vi "Dashboard Main.vi"() -> ()   [LabVIEW 2015]
uses:
  <vilib>/Utility/miscctls.llb/LVRowAndColumnTypeDef.ctl
  <vilib>/event_ctls.llb/eventvkey.ctl
  <vilib>/Rock Robotics/WPI/Dashboard/WPI_DashboardLogging Global.vi
  <vilib>/Rock Robotics/Network Tables/NT Read Numeric Array.vi
  <vilib>/Rock Robotics/Network Tables/NT Read Boolean.vi
  <vilib>/Utility/config.llb/Write Key (String).vi
  <vilib>/Utility/config.llb/Write Key (I32).vi
  <vilib>/Utility/config.llb/NI_LVConfig.lvlib
panel:
  in  "TCP":refnum<k5>
  in  "Rec Mode":enum32{"Stop", "Record", "Playback"}(radio)
  in  "Vision":u16(ring) items=["Camera Off", "USB Camera SW", "USB Camera HW", "IP Camera"]
  out "Camera IP":string
  out "Image Message":string="Timeout in Camera Communications"
  in  "Dashboard Tab":T1(tab)
  out "Voltage":dbl
  out "Current":dbl
  out "Pivot Outputs":cluster{"Numeric":dbl, "Numeric":dbl}(graph)
  out "Shooter":bool
  out "Fire":bool
  out "IntakePivot":bool
  out "IntakeRoller":bool
  out "Angle":dbl(slide) scale=-40.0..55.0
  in  "Select Auto":string(combo)
  out "NT Connection":bool
  in  "Camera Settings":T2={"Frame Rate"=30, "Compression"=30, "Size"=1} {"Frame Rate" scale=1.0..30.0; "Size" items=["640x480", "320x240", "160x120"]}
  out "MotorChart R":cluster{"Numeric":dbl, "Numeric":dbl}(graph)
  out "MotorChart L":T3(graph)
  out "MotorSliders R":cluster{"MotorSlide1":dbl, "MotorSlide2":dbl} {"MotorSlide2" scale=-1.0..1.0 scale format="%#_2e"; "MotorSlide1" scale=-1.0..1.0 scale format="%#_2e"}
  out "MotorSliders L":T4 {"MotorSlide4 2" scale=0.0..14.0 scale format="%#_2e"; "MotorSlide2" scale=-1.0..1.0 scale format="%#_2e"; "MotorSlide1" scale=-1.0..1.0 scale format="%#_2e"}
  out "JS1 Z":dbl(slide) scale=-1.0..1.0 scale format="%#_2e"
  out "JS1 Graph":cluster{"X":dbl, "Y":dbl}[](graph)
  out "JS1 Buttons":T5
  out "JS2 Z":dbl(slide) scale=-1.0..1.0 scale format="%#_2e"
  out "JS2 Graph":cluster{"X":dbl, "Y":dbl}[](graph)
  out "JS2 Buttons":T5
  out "Mode":T6(ring)=enum."Auto Disabled"
  in  "DB Camera Config":bool
  out "fps":dbl format="%#.1g"
  out "Mbps":dbl format="%#.1g"
  out "Mbps LED":bool
  in  "DB/String 9":string
  in  "DB/String 8":string
  in  "DB/String 7":string
  in  "DB/String 6":string
  in  "DB/String 5":string
  in  "DB/String 4":string
  in  "DB/String 3":string
  in  "DB/String 2":string
  in  "DB/String 1":string
  in  "DB/String 0":string
  in  "DB/Slider 0":dbl(slide) scale=0.0..5.0
  in  "DB/Slider 1":dbl(slide) scale=0.0..5.0
  in  "DB/Slider 2":dbl(slide) scale=0.0..5.0
  in  "DB/Slider 3":dbl(slide) scale=0.0..5.0
  out "DB/LED 3":bool
  out "DB/LED 2":bool
  out "DB/LED 1":bool
  out "DB/LED 0":bool
  in  "DB/Button 3":bool
  in  "DB/Button 2":bool
  in  "DB/Button 1":bool
  in  "DB/Button 0":bool caption="New Name"
  in  "Test Slider":dbl(slide) scale=0.0..100.0 scale format="%#_3g"
  in  "On/Off":bool caption="Solenoid"
  in  "Test Name":u16(ring) items=["Select the test to run..."]
  in  "Test Tree":string(tree)
  in  "Motor":cluster{"Value":dbl, "Enable":bool} {"Value" scale=-1.0..1.0 scale format="%#_3g"}
  out "Progress":T7 {"Test Progress" scale=0.0..100.0}
  in  "Rev/Fwd":cluster{"Forward":bool, "Reverse":bool}
  in  "Test Ring":u16(ring) items=["Monochrome", "Color"]
  out "Cmd Status":string
  in  "Execute Command":bool
  in  "Command Params":string[][](table)
  in  "Command Selection":i32(listbox)
  in  "CheckList":i32(listbox)
  out "Tree":string(tree)
  out "Camera Image":T8(plugin-control)
  out "Background":bool
  # "Left"
  # "Front"
  # "Right"
  # "Battery"
  # "This tab is a great place for autonomous settings and robot-specific values.\nPlace controls and indicators inside this tab and match name to\nDashboard Variables on robot. You can also delete this comment."
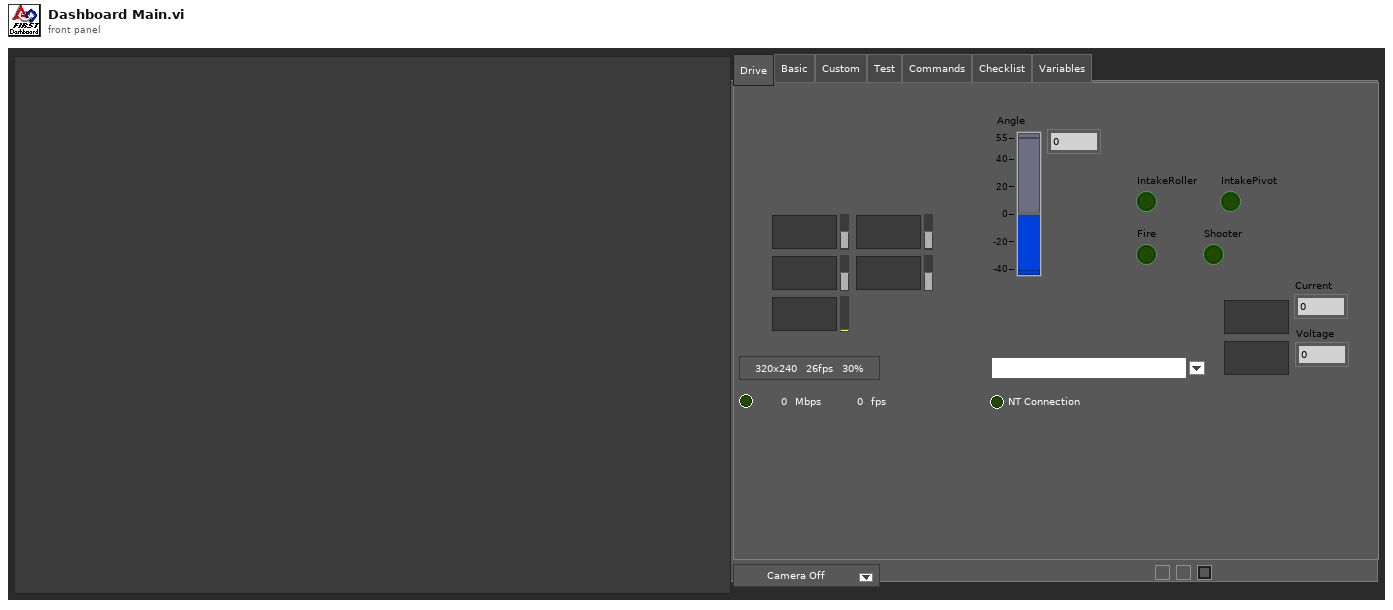
[diagram p1: front panel]
types:
  T1 = enum32{"Drive", "Basic", "Custom", "Test", "Commands", "Checklist", "Variables"}
  T2 = cluster{"Frame Rate":i32, "Compression":i32, "Size":u16}
  T3 = cluster{"Numeric":dbl, "Numeric":dbl, "Battery V":dbl}
  T4 = cluster{"MotorSlide1":dbl, "MotorSlide2":dbl, "MotorSlide4 2":dbl}
  T5 = cluster{bool, bool, bool, bool, bool, bool, bool, bool, bool, bool, bool, bool}
  T6 = enum8{"Tele-Op Disabled", "Tele-Op Enabled", "Auto Disabled", "Auto Enabled", "Test Disabled", "Test Enabled", "Disconnected", "No Code", "E-Stop"}
  T7 = cluster{"Test Progress":u8, "Test Progress Text":string}
  T8 = typedef "IMAQ Image.ctl" = refnum<image>
  T9 = cluster{"IDs":cluster{"RPC field ID":u16, "Unique ID":u16}, "String":string}
  T10 = enum32{"Drive", "Basic", "Custom", "Test", "Checklist", "Variables"}
  T11 = typedef "Image Type" = u32
  T12 = cluster{"Camera Image":refnum<vi>, "Dashboard Tab":refnum<vi>, "Background":refnum<vi>, "Vision":refnum<vi>, "Rec Mode":refnum<vi>, "Test Slider":refnum<vi>, "On/Off ":refnum<vi>, "Test Ring":refnum<vi>, "Rev/Fwd":refnum<vi>, "Test Name":refnum<vi>, "Motor":refnum<vi>, "Progress":refnum<vi>, "CheckList":refnum<vi>, "Tree":refnum<vi>, "Test Tree":refnum<vi>, "Command Params":refnum<vi>, "Command Selection":refnum<vi>, "Execute Command":refnum<vi>, "Cmd Status":refnum<vi>}
  T13 = cluster{"Error Strings":string, "Disable Counts":cluster{u16, u16}, "Rail Faults":cluster{u16, u16, u16}, "Robot IP":string, "DB Mode":u8, "Event Info":cluster{"Name":string, "Type":u8, "Number":u16, "Replay":u8}, "Camera Addr":string}
  T14 = cluster{"Storage":cluster{"Disk Free":u64, "RAM Block":u32, "RAM free":u32}, "CPU Utilization":cluster{"CPU % ISR":sgl, "CPU % Time Crit":sgl, "CPU % Timed Str":sgl, "CPU % High":sgl, "CPU % Above":sgl, "CPU % Normal":sgl, "CPU % Low":sgl}, "CAN":cluster{"% Bus Utilization":sgl, "Bus Off Cnt":u32, "TX_FIFO Full Cnt":u32, "Receive Error Cnt":u8, "Transmit Error Cnt":u8}, "HID":cluster{"HID Outputs":u32, "Rumble Low":u16, "Rumble High":u16}[]}
  T15 = cluster{"Status bits":cluster{"Test Mode":bool, "Autonomous":bool, "Enabled":bool, "Code Start":bool, "Brownout":bool, "Reserved 2":bool, "Reserved 3":bool, "E-Stop":bool}, "Code Trace":cluster{"Disabled":bool, "TeleOp":bool, "Auto":bool, "Test":bool}, "Controller Type":enum16{"unknown", "cRIO", "roboRio"}, "Code?":enum16{"unknown", "noCode", "code"}, "Battery V":dbl}
  T16 = cluster{"Control Bits":cluster{"TestMode":bool, "Autonomous":bool, "Enabled":bool, "FMS Present":bool, bool, bool, bool, "E-Stop":bool}, "Team Station ":u8, "Countdown":sgl, "Joystick Values":cluster{"Axes":dbl[], "Buttons":bool[], "POVs":i16[]}[]}
  T17 = cluster{"Axes":dbl[], "Buttons":bool[], "POVs":i16[]}[]
  T18 = cluster{"Axes":dbl[], "Buttons":bool[], "POVs":i16[]}
  T19 = cluster{"Buttons[0]":bool, "Buttons[1]":bool, "Buttons[2]":bool, "Buttons[3]":bool, "Buttons[4]":bool, "Buttons[5]":bool, "Buttons[6]":bool, "Buttons[7]":bool, "Buttons[8]":bool, "Buttons[9]":bool, "Buttons[10]":bool, "Buttons[11]":bool}
  T20 = typedef "NI_LVConfig.lvlib/Config Data RefNum.ctl" = refnum<k1>
  T21 = cluster{"Operation":enum16{"Update", "Clear"}, "Color Box":u32}[]
  T22 = typedef "eventvkey.ctl" = enum16{"ASCII", "Enter", "Return", "Shift", "Ctrl", "Alt", "Cmd", "Opt", "Caps", "NumLock", "Clear", "Break", "Up", "Down", "Left", "Right", "Insert", "Delete", "Home", "End", "PageUp", "PageDown", "Escape", "Help", "Pause", "ScrollLock", "F1", "F2", "F3", "F4", "F5", "F6", "F7", "F8", "F9", "F10", "F11", "F12", "F13", "F14", "F15", "F16", "F17", "F18", "F19", "F20", "F21", "F22", "F23", "F24", "Play", "VolumeUp", "VolumeDown", "Mute", "Two Byte Char"}
  T23 = cluster{"Image Size":bool, "Image Type":bool, "Pixel Value":bool, "ROI Information":bool, "Zoom Factor":bool}
  T24 = enum8{"Enabled", "Disabled", "Disabled and Grayed Out"}
  T25 = cluster{"Operation":enum16{"Update", "Clear"}, "Color Box":u32}
  T26 = typedef "LVRowAndColumnTypeDef.ctl" = cluster{"Row":i32, "Column":i32}
  T27 = cluster{"Shift":bool, "Ctrl":bool, "Alt":bool, "Cmd":bool, "Opt":bool}
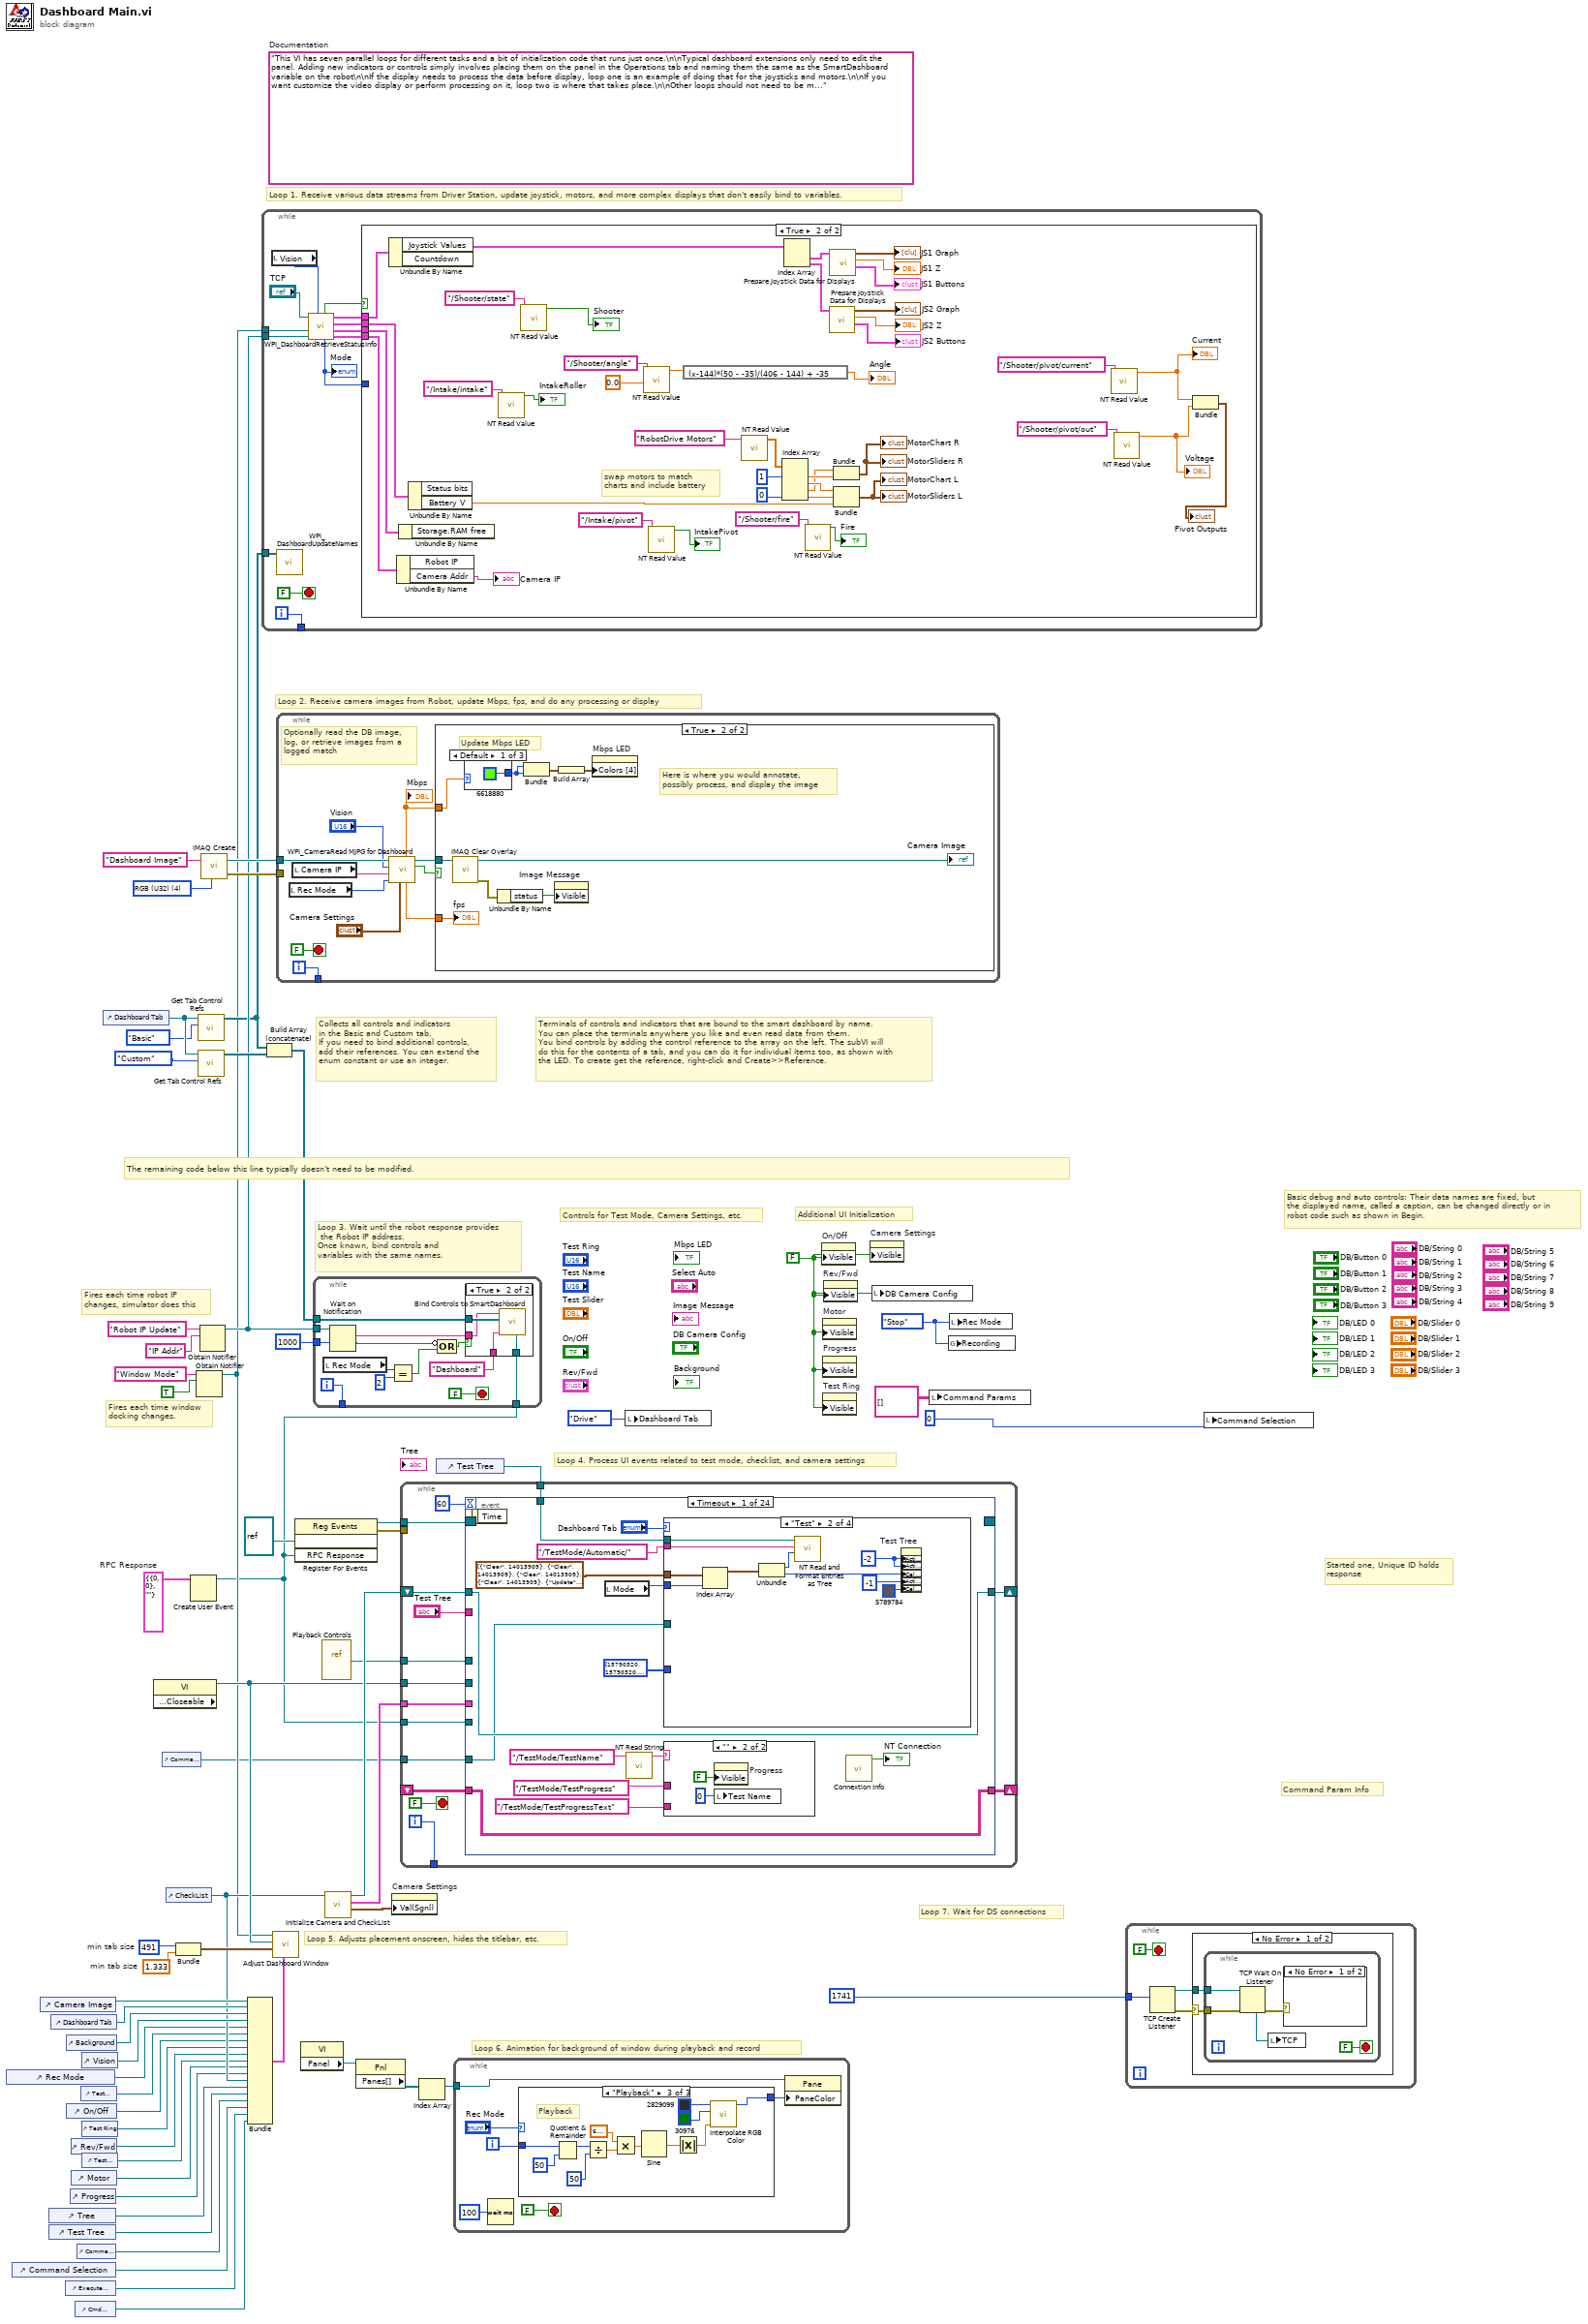
[diagram p0: block diagram]
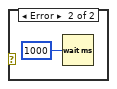
[diagram p2: hidden frame]
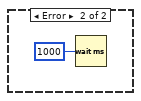
[diagram p3: hidden frame]
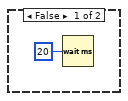
[diagram p4: hidden frame]
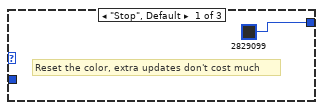
[diagram p5: hidden frame]
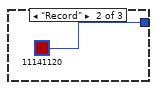
[diagram p6: hidden frame]
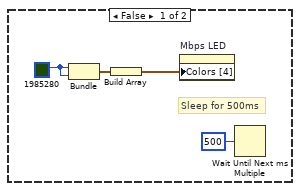
[diagram p8: hidden frame]
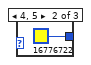
[diagram p9: hidden frame]
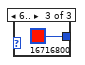
[diagram p10: hidden frame]
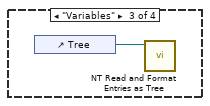
[diagram p12: hidden frame]
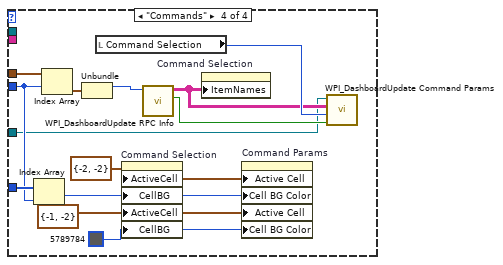
[diagram p13: hidden frame]
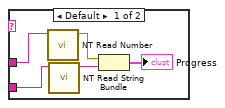
[diagram p14: hidden frame]
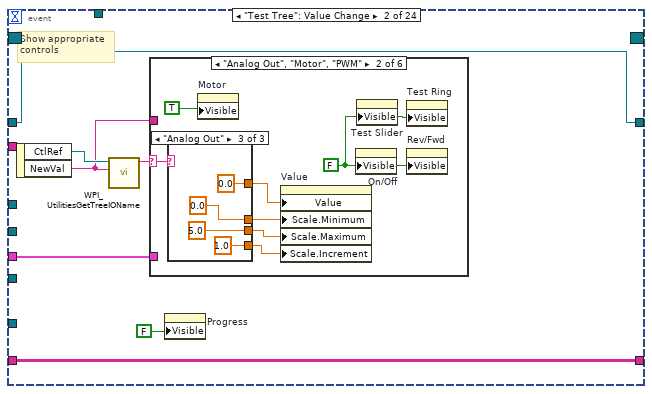
[diagram p15: hidden frame]
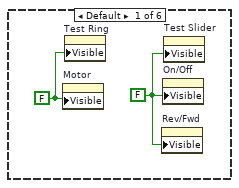
[diagram p16: hidden frame]
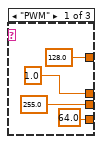
[diagram p17: hidden frame]
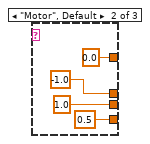
[diagram p18: hidden frame]
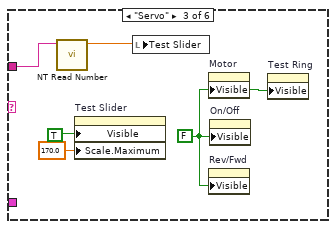
[diagram p19: hidden frame]
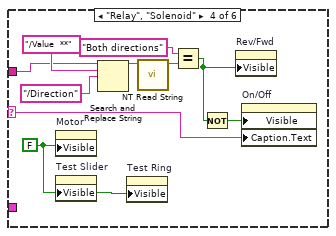
[diagram p20: hidden frame]
diagram:
  w7 = T9 {"IDs"={"RPC field ID"=0, "Unique ID"=0}, "String"=""}  # RPC Response
  w33 = 491  # min tab size
  w32 = 1.333  # min tab size
  w41 = enum32{"Stop", "Record", "Playback"}."Stop" ("Rec Mode")
  w15 = FALSE ("Visible")
  (unwired) "This VI has seven parallel loops for different tasks and a bit of initialization code that runs just once.\n\nTypical dashboard extensions only need to edit the panel. Adding new indicators or controls simply involves placing them on the panel in the Operations tab and naming them the same as the SmartDashboard variable on the robot\n\nIf the display needs to process the data before display, loop one is an example of doing that for the joysticks and motors.\n\nIf you want customize the video display or perform processing on it, loop two is where that takes place.\n\nOther loops should not need to be modified. They are pretty standard, and document the task they perform."  # Documentation
  w61 = T11 4 items=["Grayscale (U8)", "Grayscale (I16)", "Grayscale (SGL)", "Complex (CSG)", "RGB (U32)", "HSL (U32)", "RGB (U64)"] ("Image Type")
  # "Command Param Info"
  # "Started one, Unique ID holds\nresponse"
  # "Loop 7. Wait for DS connections"
  # "Basic debug and auto controls: Their data names are fixed, but\nthe displayed name, called a caption, can be changed directly or in\nrobot code such as shown in Begin."
  # "Controls for Test Mode, Camera Settings, etc."
  # "Additional UI Initialization"
  # "Loop 6. Animation for background of window during playback and record"
  # "Fires each time robot IP\nchanges, simulator does this"
  # "Fires each time window\ndocking changes."
  # "Collects all controls and indicators\nin the Basic and Custom tab.\nIf you need to bind additional controls,\nadd their references. You can extend the\nenum constant or use an integer."
  # "The remaining code below this line typically doesn't need to be modified."
  # "Loop 4. Process UI events related to test mode, checklist, and camera settings"
  # "Terminals of controls and indicators that are bound to the smart dashboard by name.\nYou can place the terminals anywhere you like and even read data from them.\nYou bind controls by adding the control reference to the array on the left. The subVI will\ndo this for the contents of a tab, and you can do it for individual items too, as shown with\nthe LED. To create get the reference, right-click and Create>>Reference."
  # "Loop 3. Wait until the robot response provides\n the Robot IP address.\nOnce known, bind controls and\nvariables with the same names."
  # "Loop 5. Adjusts placement onscreen, hides the titlebar, etc."
  # "Loop 1. Receive various data streams from Driver Station, update joystick, motors, and more complex displays that don't easily bind to variables."
  # "Loop 2. Receive camera images from Robot, update Mbps, fps, and do any processing or display"
  n1 = control-ref of="Rec Mode"() -> (w21:refnum<vi>)
  n2 = control-ref of="Command Selection"() -> (w6:refnum<vi>)
  n3 = control-ref of="Camera Image"() -> (w36:refnum<vi>)
  n4 = control-ref of="Tree"() -> (w25:refnum<vi>)
  n5 = control-ref of="Test Tree"() -> (w24:refnum<vi>)
  n6 = control-ref of="Dashboard Tab"() -> (w35:refnum<vi>)
  n7 = control-ref of="Execute Command"() -> (w8:refnum<vi>)
  n8 = control-ref of="Background"() -> (w30:refnum<vi>)
  n9 = control-ref of="On/Off"() -> (w19:refnum<vi>)
  n10 = control-ref of="Progress"() -> (w16:refnum<vi>)
  n11 = control-ref of="Rev/Fwd"() -> (w17:refnum<vi>)
  n12 = control-ref of="Motor"() -> (w22:refnum<vi>)
  n13 = control-ref of="Cmd Status"() -> (w2:refnum<vi>)
  n14 = control-ref of="Command Params"() -> (w9:refnum<vi>)
  n15 = control-ref of="Test Slider"() -> (w20:refnum<vi>)
  n16 = control-ref of="Vision"() -> (w34:refnum<vi>)
  n17 = control-ref of="Test Ring"() -> (w18:refnum<vi>)
  n18 = control-ref of="Test Name"() -> (w23:refnum<vi>)
  n19 = control-ref of="Dashboard Tab"() -> (w39:refnum<vi>)
  n20 = property class="VI" props=["Front Panel.Closeable"]() -> (reference out=w40:refnum<vi>)  [unwired: 2 in, 2 out]
  n21 = control-ref of="Command Params"() -> (w1:refnum<vi>)
  n22 = control-ref of="CheckList"() -> (w26:refnum<vi>)
  n23 = Bundle("min tab size"=w33, "min tab size"=w32) -> (w31:cluster{"min tab size":i32, "min tab size":dbl})  [unwired: 1 in]
  n24 = Create User Event(user event datatype=w7) -> (user event=w3:refnum<user-event>)  [unwired: 1 in, 1 out]
  n25 = Obtain Notifier(name (unnamed)="Window Mode", notification data type=TRUE) -> (notifier out=w12:refnum<notifier>)  [unwired: 2 in, 2 out]
  n26 = call <vilib>:"Get Tab Control Refs.vi"("Page Index"=T10."Basic" ("Dashboard Tab"), "TabControl in"=w39) -> ("ControlsOnPage"=w13:refnum<vi>[])  [unwired: 9 in]
  n27 = call <vilib>:"Get Tab Control Refs.vi"("Page Index"=T10."Custom" ("Dashboard Tab"), "TabControl in"=w39) -> ("ControlsOnPage"=w38:refnum<vi>[])  [unwired: 9 in]
  n28 = Obtain Notifier(name (unnamed)="Robot IP Update", notification data type="IP Addr" ("name (unnamed)")) -> (notifier out=w14:refnum<notifier>)  [unwired: 2 in, 2 out]
  n29 = call "IMAQ Create"("Image Name"="Dashboard Image", "Image Type"=w61) -> ("New Image"=w59:T8, "error out"=w58:errorcluster)  [unwired: 2 in, 1 out]
  n30 = Bundle("Camera Image"=w36, "Dashboard Tab"=w35, "Background"=w30, "Vision"=w34, "Rec Mode"=w21, "Test Slider"=w20, "On/Off"=w19, "Test Ring"=w18, "Rev/Fwd"=w17, "Test Name"=w23, "Motor"=w22, "Progress"=w16, "CheckList"=w26, "Tree"=w25, "Test Tree"=w24, "Command Params"=w9, "Command Selection"=w6, "Execute Command"=w8, "Cmd Status"=w2) -> (w27:T12)  [unwired: 1 in]
  n31 = while {
    tunnel: [w73] -> _
    tunnel: w14 -> [w67]
    tunnel: w13 -> [w66]
    tunnel: w12 -> [w62]
    i -> [w73]
    stop <- FALSE stop-if-true
    n32 = local read "Vision"() -> (w64:u16)
    n33 = call <vilib>:"WPI_DashboardUpdateNames.vi"("Controls on Tab"=w66) -> ()  [unwired: 11 in]
    n34 = call <vilib>:"WPI_DashboardRetrieveStatusInfo.vi"("Vision"=w64, "Binding Refnum"=w67, "Window Mode Notifier"=w62, "TCP Cnx"="TCP") -> ("Power and Errors"=w68:T13, "Robot Metrics"=w71:T14, "Status Info"=w72:T15, "Control Info"=w69:T16, "Robot Mode"=w65:T6, "Process?"=w70:bool)  [unwired: 2 in]
    "Mode" <- w65
    n35 = case shown="True" w70 {
      tunnel: w72 -> [_ w117]
      tunnel: w71 -> [_ w116]
      tunnel: w69 -> [_ w115]
      tunnel: w68 -> [_ w114]
      tunnel: w65 -> [_ _]
      frame False {
        n36 = Wait (ms)(milliseconds to wait=u32 20) -> ()  [unwired: 1 out]
      }
      frame True {
        # "swap motors to match\ncharts and include battery"
        n37 = Unbundle By Name(w115) -> ("Joystick Values"=w104:T17)  [unwired: 1 out]
        n38 = Unbundle By Name(w114) -> ("Camera Addr"=→"Camera IP":string)  [unwired: 1 out]
        n39 = Unbundle By Name(w116) -> ()  [unwired: 1 out]
        n40 = Unbundle By Name(w117) -> ("Battery V"=w105:dbl)  [unwired: 1 out]
        n41 = call-poly <vilib>:"NT Read Value.vi"("Name"="/Intake/intake") -> ("Boolean"=→"IntakeRoller":bool)  [unwired: 9 in, 1 out]
        n42 = call-poly <vilib>:"NT Read Value.vi"("Name"="/Shooter/state") -> ("Boolean"=→"Shooter":bool)  [unwired: 9 in, 1 out]
        n43 = call-poly <vilib>:"NT Read Value.vi"("Default Value"=0.0, "Name"="/Shooter/angle") -> ("Numeric"=w89:dbl)  [unwired: 8 in, 1 out]
        n44 = call-poly <vilib>:"NT Read Value.vi"("Name"="/Intake/pivot") -> ("Boolean"=→"IntakePivot":bool)  [unwired: 9 in, 1 out]
        n45 = expression code="(x-144)*(50 - -35)/(406 - 144) + -35"(w89) -> (→"Angle":dbl)
        n46 = call-poly <vilib>:"NT Read Value.vi"("Name"="RobotDrive Motors") -> ("Numeric Array"=w93:dbl[])  [unwired: 9 in, 1 out]
        n47 = Index Array(array=w93, index #1=1, index #4=0) -> (element #1=w109:dbl, element #2=w110:dbl, element #3=w108:dbl, element #4=w113:dbl)  [unwired: 2 in]
        n48 = Index Array(array=w104) -> (element #1=w103:T18, element #2=w98:T18)  [unwired: 2 in]
        n49 = call-poly <vilib>:"NT Read Value.vi"("Name"="/Shooter/fire") -> ("Boolean"=→"Fire":bool)  [unwired: 9 in, 1 out]
        n50 = call "Prepare Joystick Data for Displays.vi"("Joystick Values"=w98) -> ("Buttons"=→"JS2 Buttons":T19, "Z Axis"=→"JS2 Z":dbl, "Cartesian Data"=→"JS2 Graph":cluster{"X axis":dbl, "X axis":dbl}[])  [unwired: 8 in]
        n51 = call "Prepare Joystick Data for Displays.vi"("Joystick Values"=w103) -> ("Buttons"=→"JS1 Buttons":T19, "Z Axis"=→"JS1 Z":dbl, "Cartesian Data"=→"JS1 Graph":cluster{"X axis":dbl, "X axis":dbl}[])  [unwired: 8 in]
        n52 = Bundle("Numeric"=w108, "Numeric"=w109) -> (→"MotorChart R" →"MotorSliders R":cluster{"Numeric":dbl, "Numeric":dbl})  [unwired: 1 in]
        n53 = Bundle("Numeric"=w110, "Numeric"=w113, "Battery V"=w105) -> (→"MotorChart L" →"MotorSliders L":T3)  [unwired: 1 in]
        n54 = call-poly <vilib>:"NT Read Value.vi"("Name"="/Shooter/pivot/current") -> ("Numeric"=w77:dbl)  [unwired: 9 in, 1 out]
        "Current" <- w77
        n55 = call-poly <vilib>:"NT Read Value.vi"("Name"="/Shooter/pivot/out") -> ("Numeric"=w76:dbl)  [unwired: 9 in, 1 out]
        "Voltage" <- w76
        n56 = Bundle("Numeric"=w77, "Numeric"=w76) -> (→"Pivot Outputs":cluster{"Numeric":dbl, "Numeric":dbl})  [unwired: 1 in]
      }
    }
  }
  n57 = Build Array (concatenate)(w13, w38) -> (w37:refnum<vi>[])
  n58 = call "Adjust Dashboard Window.vi"("Sizing Refnums"=w27, "Size Constraints"=w31, "VI"=w40, "WIn Mode"=w12) -> ()  [unwired: 8 in]
  n59 = while {
    tunnel: w59 -> [w126]
    tunnel: w58 -> [_]
    tunnel: [w127] -> _
    i -> [w127]
    stop <- FALSE stop-if-true
    # "Optionally read the DB image,\nlog, or retrieve images from a\nlogged match"
    n60 = local read "Rec Mode"() -> (w121:enum32{"Stop", "Record", "Playback"})
    n61 = local read "Camera IP"() -> (w119:string)
    n62 = call <vilib>:"WPI_CameraRead MJPG for Dashboard.vi"("Camera Settings"="Camera Settings", "Rec Mode"=w121, "Camera IP"=w119, "Camera Mode"="Vision", "Refnum in"=w126) -> ("Active"=w124:bool, "Refnum out"=w125:T8, "FPS"=w123:dbl, "Bandwidth (Mbps)"=w118:dbl)  [unwired: 3 in]
    "Mbps" <- w118
    n63 = case shown="True" w124 {
      tunnel: w125 -> [_ w136]
      tunnel: w118 -> [_ w135]
      tunnel: w123 -> [_ w133]
      frame False {
        w129 = u32 1985280 ("Color Box")
        # "Sleep for 500ms"
        n64 = Bundle("Color Box"=w129, "Color Box"=w129) -> (w131:cluster{"Color Box":u32, "Color Box":u32})  [unwired: 1 out]
        n65 = Build Array(w131) -> (w130:cluster{"Color Box":u32, "Color Box":u32}[])
        n66 = property on="Mbps LED" class="Bool (strict)"("Colors [4]"=w130) -> ()  [unwired: 2 in, 2 out]
        n67 = Wait Until Next ms Multiple(millisecond multiple=u32 500) -> ()  [unwired: 1 out]
      }
      frame True {
        # "Here is where you would annotate,\npossibly process, and display the image"
        # "Update Mbps LED"
        n68 = call "IMAQ Clear Overlay"("Image"=w136) -> ("error out"=w140:errorcluster, "Image Out"=→"Camera Image":T8)  [unwired: 2 in, 7 out]
        n69 = case shown="Default" w135 {
          tunnel: [u32 6618880 ("Color Box") u32 16776722 ("Color Box") u32 16716800 ("Color Box")] -> w137
          frame Default {
          }
          frame 4, 5 {
          }
          frame 6.. {
          }
        }
        n70 = Unbundle By Name(w140) -> ("status"=w141:bool)
        n71 = Bundle("Color Box"=w137, "Color Box"=w137) -> (w139:cluster{"Color Box":u32, "Color Box":u32})  [unwired: 1 out]
        n72 = property on="Image Message" class="Str"("Visible"=w141) -> ()  [unwired: 2 in, 2 out]
        n73 = Build Array(w139) -> (w138:cluster{"Color Box":u32, "Color Box":u32}[])
        n74 = property on="Mbps LED" class="Bool (strict)"("Colors [4]"=w138) -> ()  [unwired: 2 in, 2 out]
        "fps" <- w133
      }
    }
  }
  n75 = register-events(refnum<vi> refnum, w3) -> (reference out=w45:refnum<event-registration>, error out=w44:errorcluster)  [unwired: 2 in]
  n76 = property class="VI"() -> ("Panel"=w48:refnum<vi>)  [unwired: 2 in, 2 out]
  n77 = while {
    tunnel: w37 -> [w157]
    tunnel: w14 -> [w155]
    tunnel: [w153] -> _
    tunnel: u32 1000 ("milliseconds to wait") -> [w152]
    tunnel: w3 -> [w145]
    i -> [w153]
    stop <- FALSE stop-if-true
    n78 = local read "Rec Mode"() -> (w148:enum32{"Stop", "Record", "Playback"})
    n79 = Wait on Notification(notifier=w155, timeout in ms (-1)=w152) -> (notification=w154:string, timed out?=w150:bool)  [unwired: 2 in, 2 out]
    n80 = Equal?(x=w148, y=u16 2 ("Rec Mode")) -> (x = y?=w149:bool)
    n81 = Compound Arithmetic op=OR(invert w150, w149) -> (w151:bool)
    n82 = case shown="True" w151 {
      tunnel: w157 -> [_ w161]
      tunnel: w154 -> [_ w160]
      tunnel: "Dashboard" -> [_ w159]
      tunnel: w145 -> [_ w158]
      frame False {
      }
      frame True {
        n83 = call <vilib>:"Bind Controls to SmartDashboard.vi"("RPC ref"=w158, "Client Name"=w159, "Bound Control Refs"=w161, "Server IP Address"=w160) -> ()  [unwired: 8 in]
      }
    }
  }
  n84 = vi-ref "Playback Controls.vi"() -> (w46:refnum<vi>)
  n85 = call "Initialize Camera and CheckList.vi"("ListBox in"=w26) -> ("Cluster"=w52:cluster{"value":i32, "value":i32, "index":i32}, "Array"=w53:cluster{string[]}[], "File Refnum"=w51:T20)  [unwired: 8 in]
  n86 = property class="Pnl"(reference=w48) -> ("Panes[]"=w49:refnum<vi>[])  [unwired: 1 in, 2 out]
  n87 = property on="Camera Settings" class="Clust (strict)"("Val(Sgnl)"=w52) -> ()  [unwired: 2 in, 2 out]
  n88 = Index Array(array=w49) -> (element=w47:refnum<vi>)  [unwired: 1 in]
  n89 = control-ref of="Test Tree"() -> (w50:refnum<vi>)
  n90 = while {
    tunnel: w53 -> [w173]
    shift-right: [w172] -> _
    shift-left: w51 -> [w171]
    tunnel: [w170] -> _
    tunnel: w50 -> [w169]
    tunnel: w46 -> [w168]
    tunnel: w45 -> [w167]
    tunnel: w44 -> [_]
    tunnel: w40 -> [w166]
    tunnel: w3 -> [w165]
    tunnel: w1 -> [w164]
    shift-right: [w163] -> _
    shift-left: _ -> [w162]
    i -> [w170]
    stop <- FALSE stop-if-true
    n91 = event shown="[0] Timeout" {
      selector: w167 -> [_ _ _ _ _ _ _ _ _ _ _ _ _ _ _ _ _ _ _ _ _ _ _ _]
      dyn-events: [_ _ _ _ _ _ _ _ _ _ _ _ _ _ _ _ _ _ w482 _ _ _ _ _] -> _
      timeout: u32 60 ("milliseconds to wait") -> [_ _ _ _ _ _ _ _ _ _ _ _ _ _ _ _ _ _ _ _ _ _ _ _]
      tunnel: w169 -> [w186 _ _ _ _ _ _ _ _ _ _ _ _ _ _ _ _ _ _ _ _ _ _ _]
      tunnel: "Test Tree" -> [_ _ _ _ _ _ _ _ _ _ _ _ _ w445 w454 w457 w462 w471 _ _ _ _ _ _]
      tunnel: w173 -> [_ w224 _ _ _ _ _ _ _ _ _ w407 w438 _ _ _ _ _ _ _ _ _ _ _]
      tunnel: [w183 w223 w327 w333 w343 w347 w353 w365 w373 w379 w392 w406 w431 w444 w452 w456 w461 w470 w484 w500 w502 w510 w521 w526] -> w172
      tunnel: w171 -> [w183 w223 w327 w333 w343 w347 w353 w365 w373 w379 w392 w405 w431 w444 w452 w456 w461 w470 w484 w500 w502 w510 w521 w526]
      tunnel: w168 -> [_ _ _ _ _ _ _ _ _ _ _ _ _ _ _ _ _ _ w485 _ w505 _ _ _]
      tunnel: w166 -> [_ _ _ _ _ _ _ _ _ _ _ _ _ _ _ _ _ _ w480 _ _ _ _ _]
      tunnel: w165 -> [_ _ _ _ _ _ _ _ _ _ _ _ _ _ _ _ _ _ w476 _ _ _ _ _]
      tunnel: w164 -> [w178 _ _ _ _ _ w351 _ _ _ _ _ _ _ _ _ _ _ _ _ _ _ _ _]
      tunnel: [w177 w222 w326 w332 w342 w348 w349 w359 w370 w378 w391 w404 w430 w443 w451 w455 w460 w469 w475 w498 w501 w506 w514 w527] -> w163
      tunnel: w162 -> [w177 w222 w326 w332 w342 w348 w349 _ _ w378 w391 w404 w430 w443 w451 w455 w460 w469 w475 w498 w501 w506 w514 w527]
      event Timeout {
        n92 = event-data() -> ()  [unwired: 1 in, 1 out]
        n93 = local read "Mode"() -> (w180:T6)
        n94 = call <vilib>:"NT Read String.vi"("Name"="/TestMode/TestName") -> ("String"=w189:string)  [unwired: 9 in, 1 out]
        n95 = case shown="\"Test\"" "Dashboard Tab" {
          tunnel: w186 -> [_ w200 _ _]
          tunnel: "/TestMode/Automatic/" ("Name Pattern") -> [_ w199 _ _]
          tunnel: T21 [{"Operation"=enum."Clear", "Color Box"=14013909}, {"Operation"=enum."Clear", "Color Box"=14013909}, {"Operation"=enum."Clear", "Color Box"=14013909}, {"Operation"=enum."Clear", "Color Box"=14013909}, {"Operation"=enum."Update", "Color Box"=14013909}, {"Operation"=enum."Update", "Color Box"=16777215}, {"Operation"=enum."Clear", "Color Box"=14013909}, {"Operation"=enum."Clear", "Color Box"=14013909}, {"Operation"=enum."Clear", "Color Box"=14013909}] -> [_ w192 _ w209]
          tunnel: w180 -> [_ w191 _ w208]
          tunnel: u32[] [15790320, 15790320, 15790320, 15790320, 16777215, 16777215, 15790320, 15790320, 15790320] -> [_ _ _ w214]
          tunnel: w178 -> [_ _ _ w202]
          frame "Custom", Default {
          }
          frame "Test" {
            w198 = -2 ("Active Item:Row Number")
            n96 = Index Array(array=w192, index=w191) -> (element=w193:T25)
            n97 = Unbundle(w193) -> ("Operation"=w194:enum16{"Update", "Clear"}, "Color Box"=w195:u32)
            n98 = call <vilib>:"NT Read and Format Entries as Tree.vi"("Operation"=w194, "Name Pattern"=w199, "Tree Refnum"=w200) -> ()  [unwired: 7 in, 2 out]
            n99 = property on="Test Tree" class="Tree (strict)"("Active Item Row Number"=w198, "ActiveColNum"=w198, "CellBG"=w195, "Active Item Row Number"=-1 ("Active Item:Row Number"), "CellBG"=u32 5789784 ("Color Box")) -> ()  [unwired: 2 in, 2 out]
          }
          frame "Variables" {
            n100 = control-ref of="Tree"() -> (w201:refnum<vi>)
            n101 = call <vilib>:"NT Read and Format Entries as Tree.vi"("Tree Refnum"=w201) -> ()  [unwired: 9 in, 2 out]
          }
          frame "Commands" {
            w210 = u32 5789784 ("Color Box")
            w211 = T26 {"Row"=-1, "Column"=-2} ("Active Cell:Active Cell")
            w213 = T26 {"Row"=-2, "Column"=-2} ("Active Cell:Active Cell")
            n102 = Index Array(array=w214, index=w208) -> (element=w212:u32)
            n103 = Index Array(array=w209, index=w208) -> (element=w207:T25)
            n104 = Unbundle(w207) -> ("Operation"=w206:enum16{"Update", "Clear"})  [unwired: 1 out]
            n105 = local read "Command Selection"() -> (w205:i32)
            n106 = property on="Command Selection" class="MCListbox (strict)"("ActiveCell"=w213, "CellBG"=w212, "ActiveCell"=w211, "CellBG"=w210) -> ()  [unwired: 2 in, 2 out]
            n107 = call <vilib>:"WPI_DashboardUpdate RPC Info.vi"("Operation"=w206) -> ("update"=w204:bool, "commands"=w203:string[][])  [unwired: 9 in]
            n108 = property on="Command Selection" class="MCListbox (strict)"("ItemNames"=w203) -> ()  [unwired: 2 in, 2 out]
            n109 = property on="Command Params" class="Tbl (strict)"("Active Cell"=w213, "Cell BG Color"=w212, "Active Cell"=w211, "Cell BG Color"=w210) -> ()  [unwired: 2 in, 2 out]
            n110 = call <vilib>:"WPI_DashboardUpdate Command Params.vi"("Update"=w204, "NewVal"=w205, "Commands"=w203, "Param Tbl"=w202) -> ()  [unwired: 7 in, 1 out]
          }
        }
        n111 = case shown="\"\"" w189 {
          tunnel: "/TestMode/TestProgress" ("Name") -> [w216 _]
          tunnel: "/TestMode/TestProgressText" ("Name") -> [w215 _]
          frame Default {
            n112 = call <vilib>:"NT Read Number.vi"("Name"=w216) -> ("Numeric"=w217:dbl)  [unwired: 9 in, 1 out]
            n113 = call <vilib>:"NT Read String.vi"("Name"=w215) -> ("String"=w218:string)  [unwired: 9 in, 1 out]
            n114 = Bundle("Numeric"=w217, "String"=w218) -> (→"Progress":cluster{"Numeric":dbl, "String":string})  [unwired: 1 in]
          }
          frame "" {
            n115 = property on="Progress" class="Clust (strict)"("Visible"=FALSE) -> ()  [unwired: 2 in, 2 out]
            n116 = local write "Test Name"(u16 0) -> ()
          }
        }
        n117 = call <vilib>:"Connextion Info.vi"() -> ("Connected"=→"NT Connection":bool)  [unwired: 10 in, 1 out]
      }
      event "Test Tree": Value Change {
        # "Show appropriate\ncontrols"
        n118 = event-data() -> ("CtlRef"=w227:refnum<vi>, "NewVal"=w225:string)  [unwired: 1 in]
        n119 = call <vilib>:"WPI_UtilitiesGetTreeIOName.vi"("NewVal"=w225, "TreeControl in"=w227) -> ("I/O Name"=w228:string)  [unwired: 9 in]
        n120 = case shown="\"Analog Out\", \"Motor\", \"PWM\"" w228 {
          selector: w228 -> [_ w235 _ w257 w266 _]
          tunnel: w225 -> [_ _ w254 w256 _ w273]
          tunnel: w224 -> [_ _ _ _ _ w272]
          frame Default {
            w230 = FALSE ("Visible")
            w229 = FALSE ("Visible")
            n121 = property on="Motor" class="Clust (strict)"("Visible"=w229) -> ()  [unwired: 2 in, 2 out]
            n122 = property on="Test Ring" class="Ring (strict)"("Visible"=w229) -> ()  [unwired: 2 in, 2 out]
            n123 = property on="Rev/Fwd" class="Clust (strict)"("Visible"=w230) -> ()  [unwired: 2 in, 2 out]
            n124 = property on="On/Off" class="Bool (strict)"("Visible"=w230) -> ()  [unwired: 2 in, 2 out]
            n125 = property on="Test Slider" class="Slide (strict)"("Visible"=w230) -> ()  [unwired: 2 in, 2 out]
          }
          frame "Analog Out", "Motor", "PWM" {
            w236 = FALSE ("Visible")
            n126 = case shown="\"Analog Out\"" w235 {
              tunnel: [1.0 ("Value") -1.0 ("Value") 0.0 ("Value")] -> w234
              tunnel: [255.0 ("Value") 1.0 ("Value") 5.0 ("Value")] -> w233
              tunnel: [128.0 ("Value") 0.0 ("Value") 0.0 ("Value")] -> w232
              tunnel: [64.0 ("Value") 0.5 ("Value") 1.0 ("Value")] -> w231
              frame "PWM" {
              }
              frame "Motor", Default {
              }
              frame "Analog Out" {
              }
            }
            n127 = property on="Motor" class="Clust (strict)"("Visible"=TRUE) -> ()  [unwired: 2 in, 2 out]
            n128 = property on="Value" class="Slide (strict)"("Value"=w232, "Scale.Minimum"=w234, "Scale.Maximum"=w233, "Scale.Increment"=w231) -> ()  [unwired: 2 in, 2 out]
            n129 = property on="On/Off" class="Bool (strict)"("Visible"=w236) -> ()  [unwired: 2 in, 2 out]
            n130 = property on="Test Slider" class="Slide (strict)"("Visible"=w236) -> ()  [unwired: 2 in, 2 out]
            n131 = property on="Test Ring" class="Ring (strict)"("Visible"=w236) -> ()  [unwired: 2 in, 2 out]
            n132 = property on="Rev/Fwd" class="Clust (strict)"("Visible"=w236) -> ()  [unwired: 2 in, 2 out]
          }
          frame "Servo" {
            w252 = FALSE ("Visible")
            n133 = call <vilib>:"NT Read Number.vi"("Name"=w254) -> ("Numeric"=w253:dbl)  [unwired: 9 in, 1 out]
            n134 = property on="Test Slider" class="Slide (strict)"("Visible"=TRUE, "Scale.Maximum"=170.0 ("Scale.Range:Maximum")) -> ()  [unwired: 2 in, 2 out]
            n135 = local write "Test Slider"(w253) -> ()
            n136 = property on="Motor" class="Clust (strict)"("Visible"=w252) -> ()  [unwired: 2 in, 2 out]
            n137 = property on="Rev/Fwd" class="Clust (strict)"("Visible"=w252) -> ()  [unwired: 2 in, 2 out]
            n138 = property on="On/Off" class="Bool (strict)"("Visible"=w252) -> ()  [unwired: 2 in, 2 out]
            n139 = property on="Test Ring" class="Ring (strict)"("Visible"=w252) -> ()  [unwired: 2 in, 2 out]
          }
          frame "Relay", "Solenoid" {
            w255 = FALSE ("Visible")
            n140 = property on="Motor" class="Clust (strict)"("Visible"=w255) -> ()  [unwired: 2 in, 2 out]
            n141 = property on="Test Slider" class="Slide (strict)"("Visible"=w255) -> ()  [unwired: 2 in, 2 out]
            n142 = Search and Replace String(input string=w256, search string="/Value  **", replace string="/Direction") -> (result string=w262:string)  [unwired: 5 in, 3 out]
            n143 = property on="Test Ring" class="Ring (strict)"("Visible"=w255) -> ()  [unwired: 2 in, 2 out]
            n144 = call <vilib>:"NT Read String.vi"("Name"=w262) -> ("String"=w260:string)  [unwired: 9 in, 1 out]
            n145 = Equal?(x="Both directions", y=w260) -> (x = y?=w258:bool)
            n146 = Not(x=w258) -> (.not. x?=w259:bool)
            n147 = property on="Rev/Fwd" class="Clust (strict)"("Visible"=w258) -> ()  [unwired: 2 in, 2 out]
            n148 = property on="On/Off" class="Bool (strict)"("Visible"=w259, "Caption.Text"=w257) -> ()  [unwired: 2 in, 2 out]
          }
          frame "Compressor", "Digital Out" {
            w265 = FALSE ("Visible")
            # "Get direction and finish"
            n149 = property on="Motor" class="Clust (strict)"("Visible"=w265) -> ()  [unwired: 2 in, 2 out]
            n150 = property on="Test Slider" class="Slide (strict)"("Visible"=w265) -> ()  [unwired: 2 in, 2 out]
            n151 = property on="Test Ring" class="Ring (strict)"("Visible"=w265) -> ()  [unwired: 2 in, 2 out]
            n152 = property on="On/Off" class="Bool (strict)"("Visible"=TRUE, "Caption.Text"=w266) -> ()  [unwired: 2 in, 2 out]
            n153 = property on="Rev/Fwd" class="Clust (strict)"("Visible"=FALSE) -> ()  [unwired: 2 in, 2 out]
          }
          frame "Camera" {
            n154 = call <vilib>:"Get Last Path Segment.vi"("String in"=w273) -> ("String out"=w274:string)  [unwired: 10 in]
            n155 = property on="On/Off" class="Bool (strict)"("Visible"=FALSE) -> ()  [unwired: 2 in, 2 out]
            n156 = property on="Motor" class="Clust (strict)"("Visible"=FALSE) -> ()  [unwired: 2 in, 2 out]
            n157 = property on="Rev/Fwd" class="Clust (strict)"("Visible"=FALSE) -> ()  [unwired: 2 in, 2 out]
            n158 = case shown="\"White Balance  **\"" w274 {
              tunnel: w273 -> [w280 w289 w298 w307 w316 _ w322]
              tunnel: w272 -> [w278 w286 w295 w304 w313 _ _]
              frame "Size  **" {
                n159 = Index Array(array=w278) -> (element=w277:cluster{string[]})  [unwired: 1 in]
                n160 = call <vilib>:"NT Read String.vi"("Name"=w280) -> ("String"=w279:string)  [unwired: 9 in, 1 out]
                n161 = Unbundle(w277) -> (w275:string[])
                n162 = Match First String(2:w275, 3:w279) -> (0:w276:i32)  [unwired: 1 out]
                n163 = property on="Test Ring" class="Ring (strict)"("Value"=w276, "Strings []"=w275) -> ()  [unwired: 2 in, 2 out]
                n164 = property on="Test Ring" class="Ring (strict)"("Visible"=TRUE) -> ()  [unwired: 2 in, 2 out]
                n165 = property on="Test Slider" class="Slide (strict)"("Visible"=FALSE) -> ()  [unwired: 2 in, 2 out]
              }
              frame "White Balance  **" {
                n166 = Index Array(array=w286, index=1) -> (element=w287:cluster{string[]})
                n167 = call <vilib>:"NT Read String.vi"("Name"=w289) -> ("String"=w288:string)  [unwired: 9 in, 1 out]
                n168 = Unbundle(w287) -> (w284:string[])
                n169 = Match First String(2:w284, 3:w288) -> (0:w283:i32)  [unwired: 1 out]
                n170 = property on="Test Ring" class="Ring (strict)"("Value"=w283, "Strings []"=w284) -> ()  [unwired: 2 in, 2 out]
                n171 = property on="Test Ring" class="Ring (strict)"("Visible"=TRUE) -> ()  [unwired: 2 in, 2 out]
                n172 = property on="Test Slider" class="Slide (strict)"("Visible"=FALSE) -> ()  [unwired: 2 in, 2 out]
              }
              frame "Exposure  **" {
                n173 = Index Array(array=w295, index=2) -> (element=w296:cluster{string[]})
                n174 = call <vilib>:"NT Read String.vi"("Name"=w298) -> ("String"=w297:string)  [unwired: 9 in, 1 out]
                n175 = Unbundle(w296) -> (w292:string[])
                n176 = Match First String(2:w292, 3:w297) -> (0:w293:i32)  [unwired: 1 out]
                n177 = property on="Test Ring" class="Ring (strict)"("Value"=w293, "Strings []"=w292) -> ()  [unwired: 2 in, 2 out]
                n178 = property on="Test Ring" class="Ring (strict)"("Visible"=TRUE) -> ()  [unwired: 2 in, 2 out]
                n179 = property on="Test Slider" class="Slide (strict)"("Visible"=FALSE) -> ()  [unwired: 2 in, 2 out]
              }
              frame "Exposure Priority  **" {
                n180 = Index Array(array=w304, index=3) -> (element=w305:cluster{string[]})
                n181 = call <vilib>:"NT Read String.vi"("Name"=w307) -> ("String"=w306:string)  [unwired: 9 in, 1 out]
                n182 = Unbundle(w305) -> (w301:string[])
                n183 = Match First String(2:w301, 3:w306) -> (0:w302:i32)  [unwired: 1 out]
                n184 = property on="Test Ring" class="Ring (strict)"("Value"=w302, "Strings []"=w301) -> ()  [unwired: 2 in, 2 out]
                n185 = property on="Test Ring" class="Ring (strict)"("Visible"=TRUE) -> ()  [unwired: 2 in, 2 out]
                n186 = property on="Test Slider" class="Slide (strict)"("Visible"=FALSE) -> ()  [unwired: 2 in, 2 out]
              }
              frame "Color Enable  **" {
                n187 = Index Array(array=w313, index=4) -> (element=w314:cluster{string[]})
                n188 = call <vilib>:"NT Read String.vi"("Name"=w316) -> ("String"=w315:string)  [unwired: 9 in, 1 out]
                n189 = Unbundle(w314) -> (w310:string[])
                n190 = Match First String(2:w310, 3:w315) -> (0:w311:i32)  [unwired: 1 out]
                n191 = property on="Test Ring" class="Ring (strict)"("Value"=w311, "Strings []"=w310) -> ()  [unwired: 2 in, 2 out]
                n192 = property on="Test Ring" class="Ring (strict)"("Visible"=TRUE) -> ()  [unwired: 2 in, 2 out]
                n193 = property on="Test Slider" class="Slide (strict)"("Visible"=FALSE) -> ()  [unwired: 2 in, 2 out]
              }
              frame Default {
                n194 = property on="Test Ring" class="Ring (strict)"("Visible"=FALSE) -> ()  [unwired: 2 in, 2 out]
                n195 = property on="Test Slider" class="Slide (strict)"("Visible"=FALSE) -> ()  [unwired: 2 in, 2 out]
              }
              frame "Brightness  **", "Color Level  **", "Compression  **", "FPS  **", "Sharpness  **" {
                n196 = call <vilib>:"NT Read Number.vi"("Name"=w322) -> ("Numeric"=w321:dbl)  [unwired: 9 in, 1 out]
                n197 = local write "Test Slider"(w321) -> ()
                n198 = property on="Test Slider" class="Slide (strict)"("Visible"=TRUE, "Scale.Maximum"=100.0 ("Scale.Range:Maximum")) -> ()  [unwired: 2 in, 2 out]
                n199 = property on="Test Ring" class="Ring (strict)"("Visible"=FALSE) -> ()  [unwired: 2 in, 2 out]
              }
            }
          }
        }
        n200 = property on="Progress" class="Clust (strict)"("Visible"=FALSE) -> ()  [unwired: 2 in, 2 out]
      }
      event "Test Name": Mouse Enter {
        # "Populate the ring with the list of tests"
        n201 = event-data() -> ()  [unwired: 1 in, 1 out]
        n202 = call <vilib>:"NT Read String Array.vi"("Name"="/TestMode/TestList") -> ("String Array"=w331:string[])  [unwired: 9 in, 1 out]
        n203 = Build Array (concatenate)("Select the test to run...", w331) -> (w330:string[])
        n204 = property on="Test Name" class="Ring (strict)"("Strings []"=w330) -> ()  [unwired: 2 in, 2 out]
      }
      event "Test Name": Value Change {
        w334 = FALSE ("Visible")
        # "Tell the robot the test name to run"
        n205 = event-data() -> ("NewVal"=w338:u16)  [unwired: 1 in]
        n206 = property on="Test Name" class="Ring (strict)"() -> ("Strings []"=w339:string[])  [unwired: 2 in, 2 out]
        n207 = local write "Progress"(T7 {"Test Progress"=0, "Test Progress Text"=""} ("Progress")) -> ()
        n208 = Index Array(array=w339, index=w338) -> (element=w337:string)
        n209 = call <vilib>:"NT Write String.vi"("String"=w337, "Name"="/TestMode/TestName") -> ()  [unwired: 9 in, 1 out]
        n210 = property on="Progress" class="Clust (strict)"("Visible"=TRUE) -> ()  [unwired: 2 in, 2 out]
        n211 = property on="Motor" class="Clust (strict)"("Visible"=w334) -> ()  [unwired: 2 in, 2 out]
        n212 = property on="Test Slider" class="Slide (strict)"("Visible"=w334) -> ()  [unwired: 2 in, 2 out]
        n213 = property on="On/Off" class="Bool (strict)"("Visible"=w334) -> ()  [unwired: 2 in, 2 out]
        n214 = property on="Rev/Fwd" class="Clust (strict)"("Visible"=w334) -> ()  [unwired: 2 in, 2 out]
        n215 = property on="Test Ring" class="Ring (strict)"("Visible"=w334) -> ()  [unwired: 2 in, 2 out]
      }
      event "Select Auto": Mouse Enter {
        # "Populate the combo box with the list of autonomous options"
        n216 = event-data() -> ()  [unwired: 1 in, 1 out]
        n217 = call <vilib>:"NT Read String Array.vi"("Name"="Auto List") -> ("String Array"=w341:string[])  [unwired: 9 in, 1 out]
        n218 = property on="Select Auto" class="CmbBox"("Strings[]"=w341) -> ()  [unwired: 2 in, 2 out]
      }
      event "Select Auto": Value Change {
        # "User modified the Auto Selection. Write to NT variable so robot knows."
        n219 = event-data() -> ("NewVal"=w345:string)  [unwired: 1 in]
        n220 = call <vilib>:"NT Write String.vi"("String"=w345, "Name"="Auto Selector") -> ()  [unwired: 9 in, 1 out]
      }
      event "Command Selection": Value Change {
        # "Get the params and show in table"
        n221 = event-data() -> ("NewVal"=w352:i32)  [unwired: 1 in]
        n222 = property on="Command Selection" class="MCListbox (strict)"() -> ("ItemNames"=w350:string[][])  [unwired: 2 in, 2 out]
        n223 = call <vilib>:"WPI_DashboardUpdate Command Params.vi"("NewVal"=w352, "Commands"=w350, "Param Tbl"=w351) -> ()  [unwired: 8 in, 1 out]
      }
      event "Execute Command": Value Change {
        # "Started one, Unique ID holds\nresponse"
        n224 = event-data() -> ()  [unwired: 1 in, 1 out]
        n225 = property on="Command Selection" class="MCListbox (strict)"() -> ("ItemNames"=w364:string[][])  [unwired: 2 in, 2 out]
        n226 = Index Array(array=w364, index (row)="Command Selection", index (col)=0) -> (element=w362:string)
        n227 = call <vilib>:"Invoke Commands.vi"("Command Params"="Command Params", "Function Name"=w362) -> ("Params"=w358:u8, "Started"=w357:bool)  [unwired: 7 in, 1 out]
        n228 = Array Subset(array="Command Params", length (row)=w358) -> (w359:string[][])  [unwired: 3 in]
        n229 = Select(t="Executing" ("Cmd Status"), s=w357, f="" ("Cmd Status")) -> (s? t:f=→"Cmd Status":string)
      }
      event "Command Selection": Double Click {
        n230 = event-data() -> ("Row"=w374:i32)  [unwired: 1 in]
        n231 = property on="Command Selection" class="MCListbox (strict)"() -> ("ItemNames"=w377:string[][])  [unwired: 2 in, 2 out]
        n232 = local read "Command Params"() -> (w372:string[][])
        n233 = Index Array(array=w377, index (row)=w374, index (col)=0) -> (element=w375:string)
        n234 = call <vilib>:"Invoke Commands.vi"("Command Params"=w372, "Function Name"=w375) -> ("Params"=w371:u8, "Started"=w366:bool)  [unwired: 7 in, 1 out]
        n235 = Array Subset(array=w372, length (row)=w371) -> (w370:string[][])  [unwired: 3 in]
        n236 = Select(t="Executing" ("Cmd Status"), s=w366, f="" ("Cmd Status")) -> (s? t:f=w367:string)
        n237 = local write "Cmd Status"(w367) -> ()
      }
      event "CheckList": Double Click {
        # "Shift clears all"
        # "Update symbols on the listbox"
        n238 = event-data() -> ("PlatMods.Shift"=w380:bool, "Row"=w382:i32)  [unwired: 1 in]
        n239 = case shown="True" w380 {
          tunnel: w382 -> [w386 _]
          tunnel: 1 -> [w385 _]
          frame False {
            n240 = property on="CheckList" class="LstBox (strict)"() -> ("Item Symbols"=w384:i32[])  [unwired: 2 in, 2 out]
            n241 = Replace Array Subset(array=w384, new element=w385, index=w386) -> (w383:i32[])
            n242 = property on="CheckList" class="LstBox (strict)"("Item Symbols"=w383) -> ()  [unwired: 2 in, 2 out]
          }
          frame True {
            w387 = 0 ("Top Row")
            n243 = property on="CheckList" class="LstBox (strict)"() -> ("Number of Rows"=w389:u32)  [unwired: 2 in, 2 out]
            n244 = Initialize Array(0, w389) -> (w388:i32[])
            n245 = property on="CheckList" class="LstBox (strict)"("Top Row"=w387, "Value"=w387, "Item Symbols"=w388) -> ()  [unwired: 2 in, 2 out]
          }
        }
      }
      event "CheckList": Key Down {
        # "Update symbols on the listbox\nLeft and right keys check and uncheck"
        n246 = event-data() -> ("VKey"=w394:T22)  [unwired: 1 in]
        n247 = case shown="\"Left\", \"Right\"" w394 {
          selector: w394 -> [w399 _]
          tunnel: eventvkey."Left" ("VKey") -> [w397 _]
          frame "Left", "Right" {
            n248 = Equal?(x=w397, y=w399) -> (x = y?=w398:bool)
            n249 = Select(t=0, s=w398, f=1) -> (s? t:f=w400:i32)
            n250 = property on="CheckList" class="LstBox (strict)"() -> ("Item Symbols"=w403:i32[])  [unwired: 2 in, 2 out]
            n251 = Replace Array Subset(array=w403, new element=w400, index="CheckList") -> (w402:i32[])
            n252 = property on="CheckList" class="LstBox (strict)"("Item Symbols"=w402) -> ()  [unwired: 2 in, 2 out]
          }
          frame Default {
          }
        }
      }
      event "DB Camera Config": Value Change {
        # "Show or hide the cluster of controls, store in ini file"
        n253 = event-data() -> ("NewVal"=w408:bool)  [unwired: 1 in]
        n254 = case shown="False" w408 {
          tunnel: w407 -> [w417 _]
          tunnel: [w410 w428] -> w406
          tunnel: w405 -> [w409 w428]
          frame False {
            w424 = "Camera"
            w427 = FALSE ("Visible")
            n255 = local read "Camera Settings"() -> (w416:T2)
            n256 = Index Array(array=w417) -> (element=w420:cluster{string[]})  [unwired: 1 in]
            n257 = Unbundle(w416) -> ("Frame Rate"=w415:i32, "Compression"=w414:i32, "Size"=w418:u16)
            n258 = Unbundle(w420) -> (w419:string[])
            n259 = Index Array(array=w419, index=w418) -> (element=w413:string)
            n260 = call-poly <vilib>:"Write Key.vi"("section"=w424, "value"=w413, "key"="Size", "refnum"=w409) -> ("refnum out"=w426:T20)  [unwired: 2 in, 5 out]
            n261 = call-poly <vilib>:"Write Key.vi"("section"=w424, "value"=w415, "key"="FrameRate", "refnum"=w426) -> ("refnum out"=w425:T20)  [unwired: 1 in, 6 out]
            n262 = property on="Camera Settings" class="Clust (strict)"("Visible"=w427) -> ()  [unwired: 2 in, 2 out]
            n263 = local write "DB Camera Config"(w427) -> ()
            n264 = call-poly <vilib>:"Write Key.vi"("section"=w424, "value"=w414, "key"="Compression", "refnum"=w425) -> ("refnum out"=w411:T20)  [unwired: 1 in, 6 out]
            n265 = call <vilib>:"Close Config Data.vi"("refnum"=w411) -> ("file path"=w412:path)  [unwired: 2 in, 8 out]
            n266 = call <vilib>:"Open Config Data.vi"("configuration file path"=w412) -> ("refnum"=w410:T20)  [unwired: 8 in, 2 out]
          }
          frame True {
            n267 = property on="Camera Settings" class="Clust (strict)"("Visible"=TRUE) -> ()  [unwired: 2 in, 2 out]
          }
        }
      }
      event "Camera Settings": Value Change {
        # "Update summary string when any elements of DB camera change"
        n268 = event-data() -> ("NewVal"=w442:T2)  [unwired: 1 in]
        n269 = Index Array(array=w438) -> (element=w437:cluster{string[]})  [unwired: 1 in]
        n270 = Unbundle(w442) -> ("Frame Rate"=w433:i32, "Compression"=w432:i32, "Size"=w435:u16)
        n271 = Unbundle(w437) -> (w436:string[])
        n272 = Index Array(array=w436, index=w435) -> (element=w434:string)
        n273 = Format Into String(format string="%s   %dfps   %d%%", w434, w433, w432) -> (resulting string=w439:string)  [unwired: 2 in, 1 out]
        n274 = Build Array(w439) -> (w440:string[])
        n275 = property on="DB Camera Config" class="Bool (strict)"("Strings [4]"=w440) -> ()  [unwired: 2 in, 2 out]
      }
      event "Motor.Enable": Value Change {
        # "When the test mode otor enable helper is set, update that\ntree row item's value"
        n276 = event-data() -> ("NewVal"=w449:bool)  [unwired: 1 in]
        n277 = Unbundle("Motor") -> ("Value"=w448:dbl)  [unwired: 1 out]
        n278 = Select(t=w448, s=w449, f=0.0) -> (s? t:f=w446:dbl)
        n279 = call <vilib>:"NT Write Number.vi"("Numeric"=w446, "Name"=w445) -> ()  [unwired: 9 in, 1 out]
      }
      event "Test Slider": Value Change {
        # "When the test mode slider helper is set, update that\ntree row item's value"
        n280 = event-data() -> ("NewVal"=w453:dbl)  [unwired: 1 in]
        n281 = call <vilib>:"NT Write Number.vi"("Numeric"=w453, "Name"=w454) -> ()  [unwired: 9 in, 1 out]
      }
      event "On/Off": Value Change {
        # "When the test mode on/off helper value is set, update that\ntree row item's value"
        n282 = event-data() -> ("NewVal"=w459:bool)  [unwired: 1 in]
        n283 = Boolean To (0,1)(Boolean=w459) -> (0, 1=w458:i16)
        n284 = call <vilib>:"NT Write Number.vi"("Numeric"=w458, "Name"=w457) -> ()  [unwired: 9 in, 1 out]
      }
      event "Rev/Fwd": Value Change {
        # "When the test mode helper value for relays is set, update that\ntree row item's value"
        n285 = event-data() -> ("NewVal.Forward"=w468:bool, "NewVal.Reverse"=w467:bool)  [unwired: 1 in]
        n286 = Boolean To (0,1)(Boolean=w468) -> (0, 1=w464:i16)
        n287 = Boolean To (0,1)(Boolean=w467) -> (0, 1=w466:i16)
        n288 = Negate(x=w466) -> (-x=w465:i16)
        n289 = Add(x=w464, y=w465) -> (x+y=w463:i16)
        n290 = call <vilib>:"NT Write Number.vi"("Numeric"=w463, "Name"=w462) -> ()  [unwired: 9 in, 1 out]
      }
      event "Test Ring": Value Change {
        # "When a test mode helper value is selected from the ring,\nset the tree item's variable to the string value"
        n291 = event-data() -> ("NewVal"=w473:u16)  [unwired: 1 in]
        n292 = property on="Test Ring" class="Ring (strict)"() -> ("Strings []"=w474:string[])  [unwired: 2 in, 2 out]
        n293 = Index Array(array=w474, index=w473) -> (element=w472:string)
        n294 = call <vilib>:"NT Write String.vi"("String"=w472, "Name"=w471) -> ()  [unwired: 9 in, 1 out]
      }
      event "Rec Mode": Value Change {
        # "Update globals for recording mode and path to read log from.\nClear when logging and let NetworkTables set path for vision to\nuse."
        n295 = event-data() -> ("NewVal"=w486:enum32{"Stop", "Record", "Playback"})  [unwired: 1 in]
        n296 = global write "WPI_DashboardLogging Global.vi" "Logging Filename"(path "") -> ()
        n297 = global write "WPI_DashboardLogging Global.vi" "Recording"(w486) -> ()
        n298 = case shown="\"Playback\"" w486 {
          tunnel: w485 -> [_ w488 w497]
          tunnel: [_ _ w496] -> w482
          tunnel: [_ _ w495] -> _
          tunnel: w480 -> [_ _ w493]
          tunnel: cluster{i32, i32} {-250, 170} -> [_ _ w492]
          tunnel: [_ _ T23 {"Image Size"=TRUE, "Image Type"=TRUE, "Pixel Value"=TRUE, "ROI Information"=TRUE, "Zoom Factor"=FALSE} ("Image Information Shown:All Elements")] -> w478
          tunnel: [_ _ TRUE ("Zoom Factor")] -> w477
          tunnel: w476 -> [_ _ w489]
          frame Default {
          }
          frame "Stop", "Record" {
            # "Place Window too"
            n299 = invoke class="VI" method="FP.Close"(reference=w488) -> (reference out=w487:refnum<vi>)  [unwired: 2 in, 2 out]
            n300 = invoke class="VI" method="Abort VI"(reference=w487) -> ()  [unwired: 2 in, 3 out]
          }
          frame "Playback" {
            n301 = call "Open Playback Panel.vi"("Offset"=w492, "DB VI Ref"=w493, "Playback in"=w497) -> ("Playback out"=w494:refnum<vi>)  [unwired: 8 in]
            n302 = register-events(w494, w489) -> (reference out=w496:refnum<event-registration>, error out=w495:errorcluster)  [unwired: 2 in]
          }
        }
        n303 = property on="Camera Image" class="ImageControl"("Image Information Shown"=w478, "Image Information Visible"=w477) -> ()  [unwired: 2 in, 2 out]
        n304 = call <vilib>:"WPI_DashboardNT Log FieldName Cache.vi"("Operation"=enum16{"Lookup/Add", "Index", "Clear"}."Clear") -> ()  [unwired: 8 in, 3 out]
      }
      event Panel Close {
        w499 = enum32{"Stop", "Record", "Playback"}."Stop" ("Rec Mode")
        # "Playback window has been closed, abort"
        n305 = event-data() -> ()  [unwired: 1 in, 4 out]
        n306 = local write "Rec Mode"(w499) -> ()
        n307 = global write "WPI_DashboardLogging Global.vi" "Recording"(w499) -> ()
      }
      event Panel Close {
        # "Abort playback window and ourself"
        n308 = event-data() -> ()  [unwired: 1 in, 4 out]
        n309 = invoke class="VI" method="FP.Close"(reference=w505) -> (reference out=w504:refnum<vi>)  [unwired: 2 in, 2 out]
        n310 = invoke class="VI" method="Abort VI"(reference=w504) -> (error out=w503:errorcluster)  [unwired: 2 in, 2 out]
        n311 = invoke class="VI" method="Abort VI"(error in=w503) -> ()  [unwired: 2 in, 3 out]
      }
      event User Event {
        n312 = event-data() -> ("IDs"=w513:cluster{"RPC field ID":u16, "Unique ID":u16}, "String"=w512:string)  [unwired: 1 in]
        n313 = Bundle("IDs"=w513, "String"=w512) -> (w511:T9)  [unwired: 1 in]
        n314 = call <vilib>:"Retrieve RPC Response.vi"("RPC Response"=w511) -> ("Output"=w508:string[][])  [unwired: 10 in]
        n315 = Build Array (concatenate)(w506, w508) -> (w507:string[][])
        n316 = local write "Command Params"(w507) -> ()
        n317 = local write "Cmd Status"("" ("Cmd Status")) -> ()
      }
      event "Vision": Value Change {
        # "Enable/Disable Compression slider.\nHW USB is hard-coded into the camera"
        n318 = event-data() -> ("NewVal"=w520:u16)  [unwired: 1 in]
        n319 = Equal?(x=w520, y=u32 2 ("milliseconds to wait")) -> (x = y?=w518:bool)
        n320 = Select(t=T24."Disabled and Grayed Out" ("Disabled"), s=w518, f=T24."Enabled" ("Disabled")) -> (s? t:f=w515:T24)
        n321 = property on="Compression" class="Slide (strict)"("DisabledEnum"=w515) -> ()  [unwired: 2 in, 2 out]
      }
      event "Tree": Double Click {
        n322 = event-data() -> ("PlatMods"=w525:T27, "Tag"=w524:string)  [unwired: 1 in]
        n323 = Unbundle(w525) -> ("Shift"=w523:bool)  [unwired: 4 out]
        n324 = Not(x=w523) -> (.not. x?=w522:bool)
        n325 = call <vilib>:"NT Update Persistence.vi"("Persistence"=w522, "Name"=w524) -> ()  [unwired: 9 in, 1 out]
      }
    }
  }
  n326 = while {
    tunnel: w47 -> [w529]
    i -> [w532]
    stop <- FALSE stop-if-true
    n327 = Wait (ms)(milliseconds to wait=u32 100) -> ()  [unwired: 1 out]
    n328 = case shown="\"Playback\"" "Rec Mode" {
      tunnel: w532 -> [_ _ w547]
      tunnel: [u32 2829099 ("Base Color") u32 11141120 ("Target Color") w536] -> w528
      frame "Stop", Default {
        # "Reset the color, extra updates don't cost much"
      }
      frame "Record" {
      }
      frame "Playback" {
        # "Playback"
        n329 = Quotient & Remainder(x=w547, y=u32 50 ("milliseconds to wait")) -> (x-y*floor(x/y)=w543:u32)  [unwired: 1 out]
        n330 = Divide(x=w543, y=u32 50 ("milliseconds to wait")) -> (x/y=w540:dbl)
        n331 = Multiply(x=6.283185307179586, y=w540) -> (x*y=w545:dbl)
        n332 = Sine(x=w545) -> (sin(x)=w544:dbl)
        n333 = Absolute Value(x=w544) -> (abs(x)=w537:dbl)
        n334 = call "Interpolate RGB Color.vi"("Proportion"=w537, "Target Color"=u32 30976, "Base Color"=u32 2829099) -> ("Result Color"=w536:u32)  [unwired: 8 in]
      }
    }
    n335 = property class="Pane"(reference=w529, "PaneColor"=w528) -> ()  [unwired: 1 in, 2 out]
  }
  n336 = local write "Dashboard Tab"(T1."Drive" ("Dashboard Tab")) -> ()
  n337 = property on="On/Off" class="Bool (strict)"("Visible"=w15) -> ()  [unwired: 2 in, 2 out]
  n338 = property on="Motor" class="Clust (strict)"("Visible"=w15) -> ()  [unwired: 2 in, 2 out]
  n339 = property on="Progress" class="Clust (strict)"("Visible"=w15) -> ()  [unwired: 2 in, 2 out]
  n340 = property on="Test Ring" class="Ring (strict)"("Visible"=w15) -> ()  [unwired: 2 in, 2 out]
  n341 = property on="Rev/Fwd" class="Clust (strict)"("Visible"=w15) -> ()  [unwired: 2 in, 2 out]
  n342 = property on="Camera Settings" class="Clust (strict)"("Visible"=w15) -> ()  [unwired: 2 in, 2 out]
  n343 = local write "DB Camera Config"(w15) -> ()
  n344 = local write "Command Params"(string[][] [] ("Command Params")) -> ()
  n345 = global write "WPI_DashboardLogging Global.vi" "Recording"(w41) -> ()
  n346 = local write "Rec Mode"(w41) -> ()
  n347 = while {
    tunnel: u16 1741 ("timeout ms (25000)") -> [w549]
    stop <- FALSE stop-if-true
    n348 = TCP Create Listener(10:w549) -> (0:w548:errorcluster, 3:w550:refnum<k5>)  [unwired: 4 in, 1 out]
    n349 = case shown="No Error" w548 {
      selector: w548 -> [w552 _]
      tunnel: w550 -> [w553 _]
      frame No Error {
        n350 = while {
          tunnel: w553 -> [w556]
          tunnel: w552 -> [w555]
          stop <- FALSE stop-if-true
          n351 = TCP Wait On Listener(8:w555, 11:w556) -> (0:w557:errorcluster, 4:w558:refnum<k5>)  [unwired: 2 in, 3 out]
          n352 = local write "TCP"(w558) -> ()
          n353 = case shown="No Error" w557 {
            frame No Error {
            }
            frame Error {
              n354 = Wait (ms)(milliseconds to wait=u32 1000) -> ()  [unwired: 1 out]
            }
          }
        }
      }
      frame Error {
        n355 = Wait (ms)(milliseconds to wait=u32 1000) -> ()  [unwired: 1 out]
      }
    }
  }
  n356 = local write "Command Selection"(u16 0 ("milliseconds to wait")) -> ()
